vi "Read handle.vi"(8 "error in (no error)":errorcluster, 11 "Synnax Writer in":refnum<class "Synnax Writer.lvclass">) -> (0 "error out":errorcluster, 2 "handle":u64, 3 "Synnax Writer out":refnum<class "Synnax Writer.lvclass">)   [LabVIEW 2026, in "synnax_clib.lvlib" / "Synnax Writer.lvclass"]
uses:
  Synnax Writer.lvclass
  Synnax Writer.lvclass/Synnax Writer.ctl
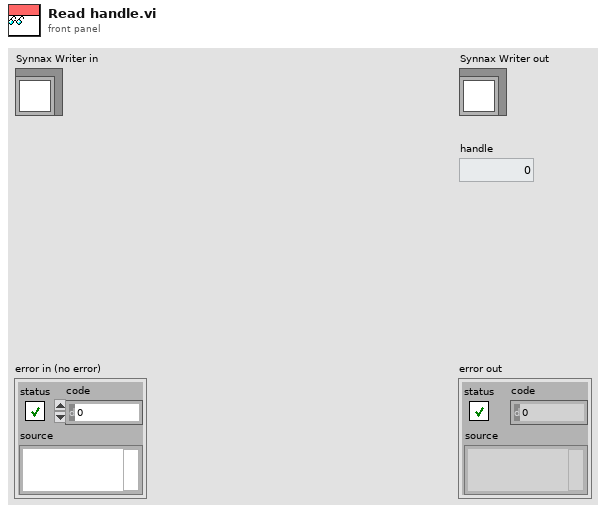
[diagram p1: front panel]
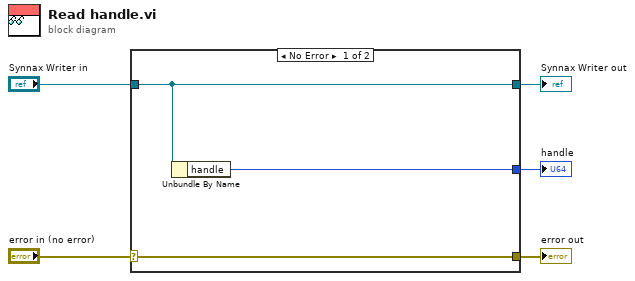
[diagram p0: block diagram]
diagram:
  n1 = case shown="No Error" "error in (no error)" {
    selector: "error in (no error)" -> [w8 w9]
    tunnel: [w8 w9] -> w4
    tunnel: [w7 w10] -> w2
    tunnel: "Synnax Writer in" -> [w7 w10]
    tunnel: [w6 _] -> w1
    frame No Error {
      n2 = Unbundle By Name(w7) -> ("handle"=w6:u64)
    }
    frame Error {
    }
  }
  "error out" <- w4
  "Synnax Writer out" <- w2
  "handle" <- w1
